vi "Finish.vi"(6 "Queues":T4, 7 "Timer parameters":refnum<vi>, 8 "Status/Errors in":refnum<vi>, 9 "Control Parameters [] in":T1[](array[typedef]) {"Aux Byte Value" format="%02x"; "Max Real Value" format="%#_6e"; "Min Real Value" format="%#_6e"; "dReal/dByte" format="%#_6e"; "Byte Value" format="%02x"; "Identifier" format="%02x"}, 10 "Main parameters in":T5={"Mode"={"Mode"=enum."Dialog", "Expert?"=FALSE, "Dialog?"=FALSE}, "Stop loop"={"Settings changed?"=FALSE, "Stop?"=refnum}, "Send message"={"Send mode"=enum."Get parameters", "Set parameter list"=0, "Get parameter list"=0, "Reset device"=0, "Length set settings message"=0, "Reset buttons?"=FALSE, "Reset Master?"=enum."General"}, "Write settings"={"Options"=enum."File 1"}, "Settings state"={"MAS locked?"=refnum, "SLV locked?"=refnum}, "Button refs"={"Stop program"=refnum, "Save settings"=refnum, "DAQ mode"=refnum, "Reset settings"=refnum, "Apply settings"=refnum, "Reset MAS"=refnum, "Reset SLV"=refnum, "Local DBase?"=refnum, "Last value DBase"=FALSE, "Database"=refnum, "Calibration"=refnum, "Save settings 2"=refnum}, "Update screen"={"Detector number"=0, "Hardware"=enum."None"}, "Files"={"Path config file"=path "", "Path def. ini file"=path "", "Path ini file 1"=path "", "Path ini file 2"=path "", "Path RBF file"=path ""}, "DB connection"={"connection reference"=refnum, "Connected?"=refnum, "ODBC Name"=""}, "Status_id"=refnum, "Time difference"=refnum, "Satellites"=refnum, "Alignment parameters"=refnum, "Page Statistics 2"=refnum, "Database"=refnum, "Page Statistics"=refnum} {"Update screen"."Detector number" format="%#.0f"; "Send message"."Reset device" format="%x"; "Send message"."Get parameter list" format="%x"; "Send message"."Set parameter list" format="%x"}, 11 "Devices in":T3) -> (0 "Status/Errors out":refnum<vi>, 1 "Control Parameters [] out":T1[](array[typedef]) {"Aux Byte Value" format="%02x"; "Max Real Value" format="%#_6e"; "Min Real Value" format="%#_6e"; "dReal/dByte" format="%#_6e"; "Byte Value" format="%02x"; "Identifier" format="%02x"}, 2 "Main parameters out":T5={"Mode"={"Mode"=enum."Dialog", "Expert?"=FALSE, "Dialog?"=FALSE}, "Stop loop"={"Settings changed?"=FALSE, "Stop?"=refnum}, "Send message"={"Send mode"=enum."Get parameters", "Set parameter list"=0, "Get parameter list"=0, "Reset device"=0, "Length set settings message"=0, "Reset buttons?"=FALSE, "Reset Master?"=enum."General"}, "Write settings"={"Options"=enum."File 1"}, "Settings state"={"MAS locked?"=refnum, "SLV locked?"=refnum}, "Button refs"={"Stop program"=refnum, "Save settings"=refnum, "DAQ mode"=refnum, "Reset settings"=refnum, "Apply settings"=refnum, "Reset MAS"=refnum, "Reset SLV"=refnum, "Local DBase?"=refnum, "Last value DBase"=FALSE, "Database"=refnum, "Calibration"=refnum, "Save settings 2"=refnum}, "Update screen"={"Detector number"=0, "Hardware"=enum."None"}, "Files"={"Path config file"=path "", "Path def. ini file"=path "", "Path ini file 1"=path "", "Path ini file 2"=path "", "Path RBF file"=path ""}, "DB connection"={"connection reference"=refnum, "Connected?"=refnum, "ODBC Name"=""}, "Status_id"=refnum, "Time difference"=refnum, "Satellites"=refnum, "Alignment parameters"=refnum, "Page Statistics 2"=refnum, "Database"=refnum, "Page Statistics"=refnum} {"Update screen"."Detector number" format="%#.0f"; "Send message"."Reset device" format="%x"; "Send message"."Get parameter list" format="%x"; "Send message"."Set parameter list" format="%x"}, 3 "Devices out":T3)   [LabVIEW 2013]
uses:
  Controls/Main_Parameters.ctl
  Controls/Mode.ctl
  Controls/Stop_Loop.ctl
  Controls/Send_Message.ctl
  Controls/Send_Message_Mode.ctl
  Controls/Master.ctl
  Controls/Write_Settings.ctl
  Controls/Write_Settings_Options.ctl
  Controls/Settings_State.ctl
  Controls/Button_Refs.ctl
  Controls/Update_Screen.ctl
  Controls/Files.ctl
  Controls/DB_Connection.ctl
  database/Connection.llb/Conn ObjectReference.ctl
  Controls/Devices.ctl
  Controls/Control_Parameters.ctl
  Controls/Queues.ctl
  Controls/One_Second.ctl
  Controls/GPS_Timestamp.ctl
  Controls/Get_Set_Connection_Options.ctl
  Controls/Get_Set_Settings_State_Options.ctl
  Controls/Get_Set_Buttons_mode.ctl
panel:
  out "Error7":errorcluster
  out "Error6":errorcluster
  out "Error5":errorcluster
  out "Error3":errorcluster
  out "Error2":errorcluster
  out "Error1":errorcluster
  out "Error4":errorcluster
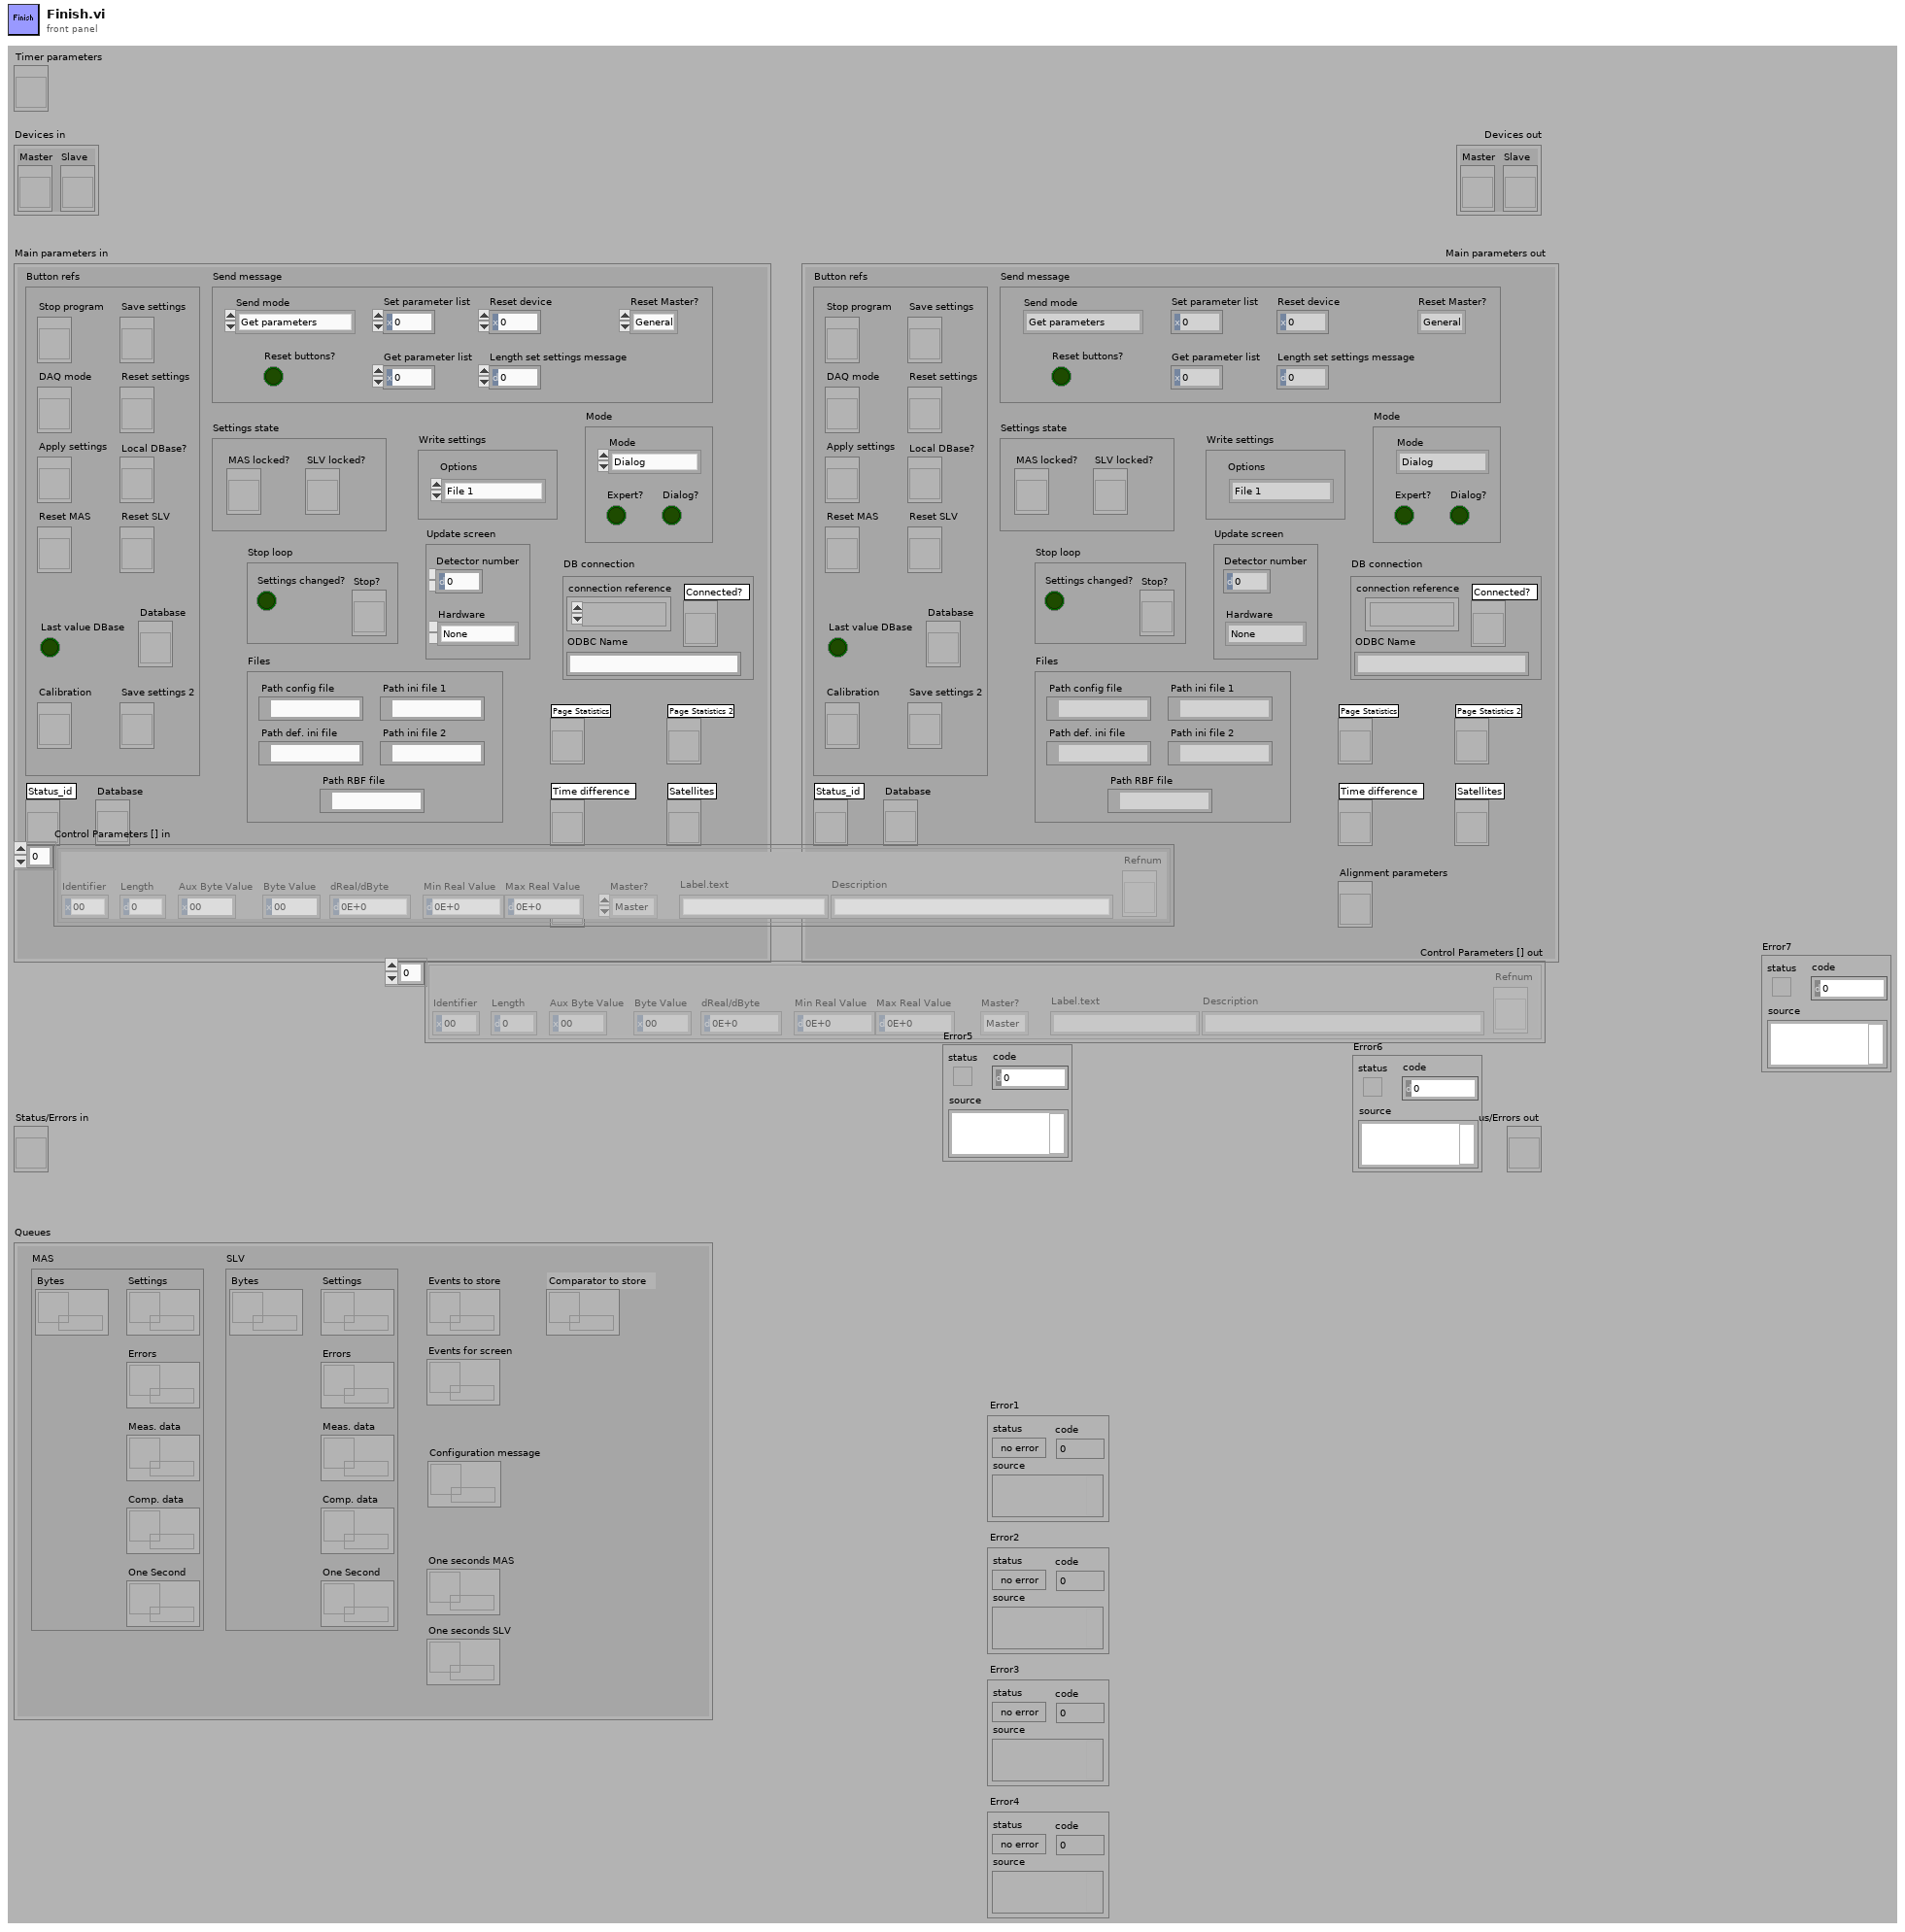
[diagram p1: front panel]
types:
  T1 = typedef "Control_Parameters.ctl" = cluster{"Identifier":u8, "Length":u16, "Byte Value":u32, "dReal/dByte":dbl, "Min Real Value":dbl, "Max Real Value":dbl, "Master?":T2, "Label.text":string, "Description":string, "Refnum":refnum<vi>, "Aux Byte Value":u32}
  T2 = typedef "Master.ctl" = enum16{"Master", "Slave", "General"}
  T3 = typedef "Devices.ctl" = cluster{"Master":refnum<vi>, "Slave":refnum<vi>}
  T4 = typedef "Queues.ctl" = cluster{"MAS":cluster{"Bytes":refnum<queue>, "Settings":refnum<queue>, "Errors":refnum<queue>, "Meas. data":refnum<queue>, "One Second":refnum<queue>, "Comp. data":refnum<queue>}, "SLV":cluster{"Bytes":refnum<queue>, "Settings":refnum<queue>, "Errors":refnum<queue>, "Meas. data":refnum<queue>, "One Second":refnum<queue>, "Comp. data":refnum<queue>}, "Events to store":refnum<queue>, "Events for screen":refnum<queue>, "One seconds MAS":refnum<queue>, "One seconds SLV":refnum<queue>, "Configuration message":refnum<queue>, "Comparator to store":refnum<queue>}
  T5 = typedef "Main_Parameters.ctl" = cluster{"Mode":T6, "Stop loop":T7, "Send message":T8, "Write settings":T10, "Settings state":T12, "Button refs":T13, "Update screen":T14, "Files":T15, "DB connection":T16, "Status_id":refnum<vi>, "Time difference":refnum<vi>, "Satellites":refnum<vi>, "Alignment parameters":refnum<vi>, "Page Statistics 2":refnum<vi>, "Database":refnum<vi>, "Page Statistics":refnum<vi>}
  T6 = typedef "Mode.ctl" = cluster{"Mode":enum8{"Stop", "Dialog", "Hisparc II", "Hisparc II DAQ", "Alignment"}, "Expert?":bool, "Dialog?":bool}
  T7 = typedef "Stop_Loop.ctl" = cluster{"Settings changed?":bool, "Stop?":refnum<vi>}
  T8 = typedef "Send_Message.ctl" = cluster{"Send mode":T9, "Set parameter list":u8, "Get parameter list":u8, "Reset device":u8, "Length set settings message":i32, "Reset buttons?":bool, "Reset Master?":T2}
  T9 = typedef "Send_Message_Mode.ctl" = enum16{"Get parameters", "Set parameters", "From front panel", "From parameters", "Reset device", "Alignment"}
  T10 = typedef "Write_Settings.ctl" = cluster{"Options":T11}
  T11 = typedef "Write_Settings_Options.ctl" = enum16{"File 1", "File 2", "Alignment", "Reset"}
  T12 = typedef "Settings_State.ctl" = cluster{"MAS locked?":refnum<vi>, "SLV locked?":refnum<vi>}
  T13 = typedef "Button_Refs.ctl" = cluster{"Stop program":refnum<vi>, "Save settings":refnum<vi>, "DAQ mode":refnum<vi>, "Reset settings":refnum<vi>, "Apply settings":refnum<vi>, "Reset MAS":refnum<vi>, "Reset SLV":refnum<vi>, "Local DBase?":refnum<vi>, "Last value DBase":bool, "Database":refnum<vi>, "Calibration":refnum<vi>, "Save settings 2":refnum<vi>}
  T14 = typedef "Update_Screen.ctl" = cluster{"Detector number":u16, "Hardware":enum8{"None", "HiSPARC I", "HiSPARC II", "HiSPARC III", "Unknown"}}
  T15 = typedef "Files.ctl" = cluster{"Path config file":path, "Path def. ini file":path, "Path ini file 1":path, "Path ini file 2":path, "Path RBF file":path}
  T16 = typedef "DB_Connection.ctl" = cluster{"connection reference":T17, "Connected?":refnum<vi>, "ODBC Name":string}
  T17 = typedef "Conn ObjectReference.ctl" = refnum<k1>
  T18 = typedef "Get_Set_Buttons_mode.ctl" = enum16{"Get", "Get DAQ", "Set", "Set settings"}
  T19 = typedef "Get_Set_Settings_State_Options.ctl" = enum16{"Get", "Lock", "Unlock"}
  T20 = typedef "Get_Set_Connection_Options.ctl" = enum16{"Get", "Set connect", "Set disconnect"}
  T21 = enum8{"Stop", "Dialog", "Hisparc II", "Hisparc II DAQ", "Alignment"}
  T22 = typedef "Semaphore RefNum" = refnum<k1>
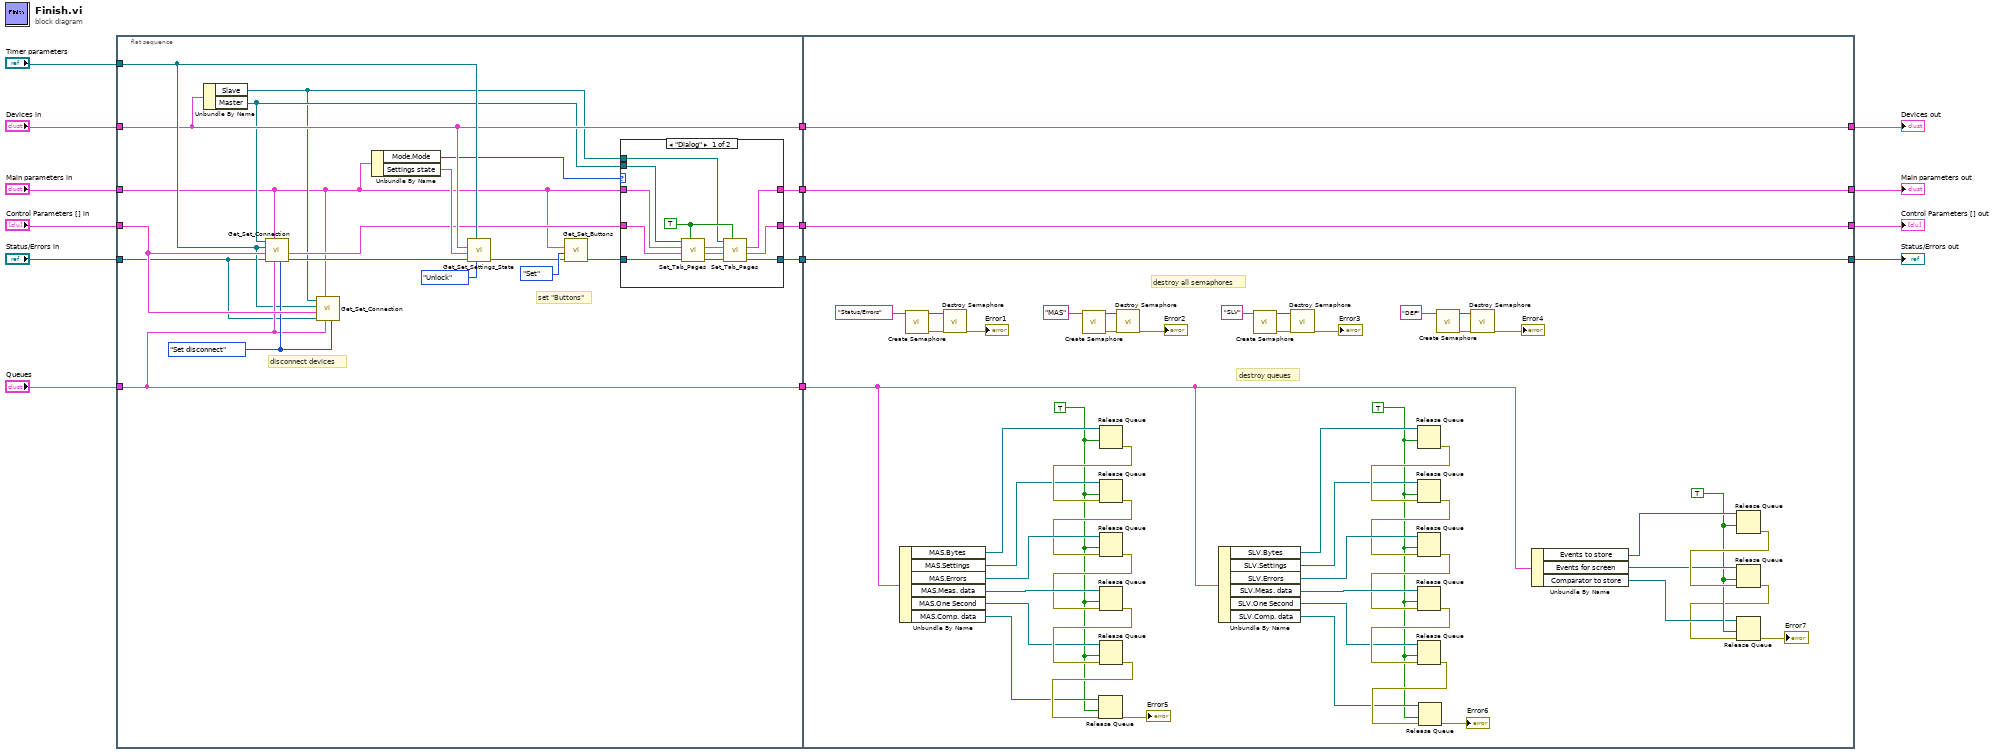
[diagram p0: block diagram]
diagram:
  n1 = flat-sequence {
    tunnel: "Timer parameters" -> [w31]
    tunnel: "Status/Errors in" -> [w27]
    tunnel: "Control Parameters [] in" -> [w35]
    tunnel: "Main parameters in" -> [w16]
    tunnel: "Devices in" -> [w29]
    tunnel: "Queues" -> [w33]
    tunnel: [w22] -> w6
    tunnel: [w29] -> w5
    tunnel: [w20] -> w4
    tunnel: [w33] -> w3
    tunnel: [w24] -> w2
    tunnel: [w102] -> w7
    tunnel: [w103] -> w8
    tunnel: [w75] -> w9
    tunnel: [w104] -> w11
    tunnel: w6 -> [w104]
    tunnel: w5 -> [w103]
    tunnel: w4 -> [w102]
    tunnel: w3 -> [w79]
    tunnel: w2 -> [w75]
    frame #0 {
      w34 = Get_Set_Connection_Options."Set disconnect" ("Get/Set")
      # "set \"Buttons\""
      # "disconnect devices"
      n2 = Unbundle By Name(w29) -> ("Slave"=w17:refnum<vi>, "Master"=w18:refnum<vi>)
      n3 = call "Get_Set_Connection.vi"("Get/Set"=w34, "Queues"=w33, "Main parameters in"=w16, "Status/Errors in"=w27, "Control Parameters [] in"=w35, "Timer parameters in"=w31, "Device in"=w18) -> ("Status/Errors out"=w32:refnum<vi>, "Control Parameters [] out"=w21:T1[])  [unwired: 3 out]
      n4 = call "Get_Set_Connection.vi"("Get/Set"=w34, "Queues"=w33, "Main parameters in"=w16, "Status/Errors in"=w27, "Control Parameters [] in"=w35, "Timer parameters in"=w31, "Device in"=w17) -> ()  [unwired: 5 out]
      n5 = Unbundle By Name(w16) -> ("Mode.Mode"=w19:T21, "Settings state"=w28:T12)
      n6 = call "Get_Set_Settings_State.vi"("Get/Set"=Get_Set_Settings_State_Options."Unlock", "Timer parameters"=w31, "Status/Errors in"=w32, "Settings state"=w28, "Devices in"=w29) -> ("Status/Errors out"=w25:refnum<vi>)  [unwired: 6 out]
      n7 = call "Get_Set_Buttons.vi"("Status/Errors in"=w25, "Set?"=Get_Set_Buttons_mode."Set", "Main parameters"=w16) -> ("Status/Errors out"=w23:refnum<vi>)  [unwired: 1 in, 7 out]
      n8 = case shown="\"Dialog\"" w19 {
        tunnel: [w41 w50] -> w24
        tunnel: w23 -> [w43 w50]
        tunnel: [w45 w49] -> w22
        tunnel: w21 -> [w47 w49]
        tunnel: [w36 w48] -> w20
        tunnel: w16 -> [w38 w48]
        tunnel: w18 -> [w40 _]
        tunnel: w17 -> [w39 _]
        frame "Dialog" {
          w44 = TRUE
          n9 = call "Set_Tab_Pages.vi"("Pages visible? (false)"=w44, "Status/Errors in"=w43, "Control Parameters [] in"=w47, "Main parameters in"=w38, "Device in"=w40) -> ("Status/Errors out"=w42:refnum<vi>, "Control Parameters [] out"=w46:T1[], "Main parameters out"=w37:T5)  [unwired: 4 out]
          n10 = call "Set_Tab_Pages.vi"("Pages visible? (false)"=w44, "Status/Errors in"=w42, "Control Parameters [] in"=w46, "Main parameters in"=w37, "Device in"=w39) -> ("Status/Errors out"=w41:refnum<vi>, "Control Parameters [] out"=w45:T1[], "Main parameters out"=w36:T5)  [unwired: 4 out]
        }
        frame Default {
        }
      }
    }
    frame #1 {
      w65 = TRUE ("force destroy? (F)")
      w67 = TRUE ("force destroy? (F)")
      w71 = TRUE ("force destroy? (F)")
      # "destroy queues"
      # "destroy all semaphores"
      n11 = Unbundle By Name(w79) -> ("MAS.Bytes"=w92:refnum<queue>, "MAS.Settings"=w93:refnum<queue>, "MAS.Errors"=w100:refnum<queue>, "MAS.Meas. data"=w99:refnum<queue>, "MAS.One Second"=w94:refnum<queue>, "MAS.Comp. data"=w72:refnum<queue>)
      n12 = call <vilib>:"Create Semaphore.vi"("name (unnamed)"="Status/Errors") -> ("error out"=w61:errorcluster, "semaphore"=w62:T22)  [unwired: 2 in, 3 out]
      n13 = call <vilib>:"Destroy Semaphore.vi"("error in (no error)"=w61, "semaphore"=w62) -> ("error out"=→"Error1":errorcluster)  [unwired: 5 out]
      n14 = call <vilib>:"Create Semaphore.vi"("name (unnamed)"="MAS") -> ("error out"=w59:errorcluster, "semaphore"=w58:T22)  [unwired: 2 in, 3 out]
      n15 = Release Queue(queue=w92, force destroy? (F)=w71) -> (error out=w98:errorcluster)  [unwired: 1 in, 2 out]
      n16 = Release Queue(queue=w93, force destroy? (F)=w71, error in (no error)=w98) -> (error out=w97:errorcluster)  [unwired: 2 out]
      n17 = Release Queue(queue=w100, force destroy? (F)=w71, error in (no error)=w97) -> (error out=w96:errorcluster)  [unwired: 2 out]
      n18 = Release Queue(queue=w99, force destroy? (F)=w71, error in (no error)=w96) -> (error out=w95:errorcluster)  [unwired: 2 out]
      n19 = Release Queue(queue=w94, force destroy? (F)=w71, error in (no error)=w95) -> (error out=w73:errorcluster)  [unwired: 2 out]
      n20 = Release Queue(queue=w72, force destroy? (F)=w71, error in (no error)=w73) -> (error out=→"Error5":errorcluster)  [unwired: 2 out]
      n21 = call <vilib>:"Destroy Semaphore.vi"("error in (no error)"=w59, "semaphore"=w58) -> ("error out"=→"Error2":errorcluster)  [unwired: 5 out]
      n22 = Unbundle By Name(w79) -> ("SLV.Bytes"=w83:refnum<queue>, "SLV.Settings"=w84:refnum<queue>, "SLV.Errors"=w91:refnum<queue>, "SLV.Meas. data"=w90:refnum<queue>, "SLV.One Second"=w85:refnum<queue>, "SLV.Comp. data"=w68:refnum<queue>)
      n23 = call <vilib>:"Create Semaphore.vi"("name (unnamed)"="SLV") -> ("error out"=w54:errorcluster, "semaphore"=w56:T22)  [unwired: 2 in, 3 out]
      n24 = call <vilib>:"Destroy Semaphore.vi"("error in (no error)"=w54, "semaphore"=w56) -> ("error out"=→"Error3":errorcluster)  [unwired: 5 out]
      n25 = Release Queue(queue=w83, force destroy? (F)=w67) -> (error out=w89:errorcluster)  [unwired: 1 in, 2 out]
      n26 = Release Queue(queue=w84, force destroy? (F)=w67, error in (no error)=w89) -> (error out=w88:errorcluster)  [unwired: 2 out]
      n27 = Release Queue(queue=w91, force destroy? (F)=w67, error in (no error)=w88) -> (error out=w87:errorcluster)  [unwired: 2 out]
      n28 = Release Queue(queue=w90, force destroy? (F)=w67, error in (no error)=w87) -> (error out=w86:errorcluster)  [unwired: 2 out]
      n29 = Release Queue(queue=w85, force destroy? (F)=w67, error in (no error)=w86) -> (error out=w69:errorcluster)  [unwired: 2 out]
      n30 = Release Queue(queue=w68, force destroy? (F)=w67, error in (no error)=w69) -> (error out=→"Error6":errorcluster)  [unwired: 2 out]
      n31 = call <vilib>:"Create Semaphore.vi"("name (unnamed)"="DEF") -> ("error out"=w52:errorcluster, "semaphore"=w53:T22)  [unwired: 2 in, 3 out]
      n32 = call <vilib>:"Destroy Semaphore.vi"("error in (no error)"=w52, "semaphore"=w53) -> ("error out"=→"Error4":errorcluster)  [unwired: 5 out]
      n33 = Unbundle By Name(w79) -> ("Events to store"=w80:refnum<queue>, "Events for screen"=w81:refnum<queue>, "Comparator to store"=w64:refnum<queue>)
      n34 = Release Queue(queue=w80, force destroy? (F)=w65) -> (error out=w82:errorcluster)  [unwired: 1 in, 2 out]
      n35 = Release Queue(queue=w81, force destroy? (F)=w65, error in (no error)=w82) -> (error out=w63:errorcluster)  [unwired: 2 out]
      n36 = Release Queue(queue=w64, force destroy? (F)=w65, error in (no error)=w63) -> (error out=→"Error7":errorcluster)  [unwired: 2 out]
    }
  }
  "Main parameters out" <- w7
  "Devices out" <- w8
  "Control Parameters [] out" <- w11
  "Status/Errors out" <- w9
